vi "1.4 Steering Encoder Deal With Skip.vi"(1 "Steering Center":bool, 2 "Steer Encoder A":bool, 3 "Steer Encoder B":bool) -> (0 "Magic Number":i32)   [LabVIEW 2011]
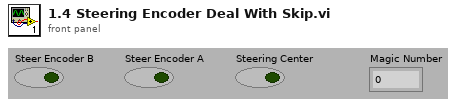
[diagram p1: front panel]
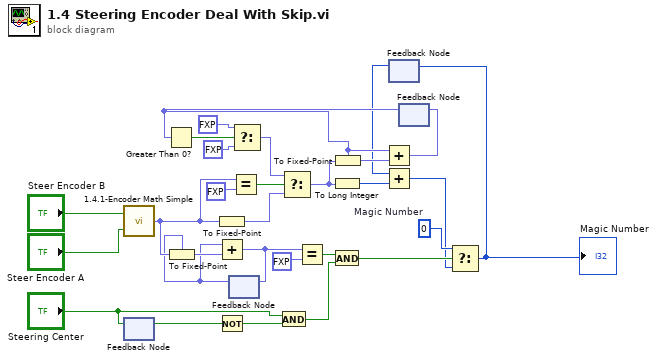
[diagram p0: block diagram]
diagram:
  w5 = 0  # Magic Number
  n1 = call "1.4.1-Encoder Math Simple.vi"("B"="Steer Encoder A", "A"="Steer Encoder B") -> ("Numeric"=w22:fxp<+/-,2,2>)
  n2 = feedback #1() -> (w7:bool)  [unwired: 1 in]
  n3 = feedback-in #1("Steering Center") -> ()
  n4 = To Fixed-Point(number=w22) -> (fixed-point=w23:fxp<+/-,3,3>)  [unwired: 1 in]
  n5 = Not(x=w7) -> (.not. x?=w6:bool)
  n6 = feedback #2() -> (w8:fxp<+/-,4,4>)  [unwired: 1 in]
  n7 = To Fixed-Point(fixed-point type=w8, number=w22) -> (fixed-point=w9:fxp<+/-,4,4>)
  n8 = Add(x=w8, y=w9) -> (x+y=w10:fxp<+/-,4,4>)
  n9 = feedback-in #2(w10) -> ()
  n10 = Equal?(x=w22, y=fxp<+/-,2,2> -2.0) -> (x = y?=w21:bool)
  n11 = And(x="Steering Center", y=w6) -> (x .and. y?=w12:bool)
  n12 = Equal?(x=w10, y=fxp<+/-,4,4> -8.0) -> (x = y?=w13:bool)
  n13 = And(x=w13, y=w12) -> (x .and. y?=w14:bool)
  n14 = feedback #3() -> (w1:i32)  [unwired: 1 in]
  n15 = feedback #4() -> (w28:fxp<+/-,4,4>)  [unwired: 1 in]
  n16 = Greater Than 0?(x=w28) -> (x > 0?=w29:bool)
  n17 = Select(t=fxp<+/-,3,3> 2.0 ("y"), s=w29, f=fxp<+/-,3,3> -2.0 ("y")) -> (s? t:f=w25:fxp<+/-,3,3>)
  n18 = Select(t=w25, s=w21, f=w23) -> (s? t:f=w24:fxp<+/-,3,3>)
  n19 = To Long Integer(number=w24) -> (32bit integer=w2:i32)
  n20 = To Fixed-Point(fixed-point type=w28, number=w24) -> (fixed-point=w19:fxp<+/-,4,4>)
  n21 = Add(x=w28, y=w19) -> (x+y=w18:fxp<+/-,4,4>)
  n22 = Add(x=w1, y=w2) -> (x+y=w4:i32)
  n23 = feedback-in #4(w18) -> ()
  n24 = Select(t=w5, s=w14, f=w4) -> (s? t:f=w3:i32)
  "Magic Number" <- w3
  n25 = feedback-in #3(w3) -> ()
